vi "LineController Analogue init v3.0.vi"(0 "lines":tag="Dev2/ao0", 1 "Power level (0-1)":dbl=1.0 min=0.0 max=1.0, 3 "error in":errorcluster, 4 "Level at max (0-5V)":dbl=5.0 min=0.0 max=5.0 step=0.05) -> (5 "task out":refnum<k21>, 6 "Gauge":dbl(knob) scale=0.0..5.0, 7 "error out":errorcluster)   [LabVIEW 2014]
uses:
  <vilib>/DAQmx/create/channels.llb/DAQmx Create Channel (AO-Voltage-Basic).vi
  <vilib>/DAQmx/write.llb/DAQmx Write (Analog DBL 1Chan 1Samp).vi
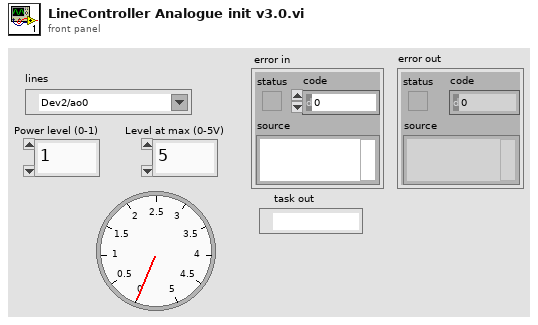
[diagram p1: front panel]
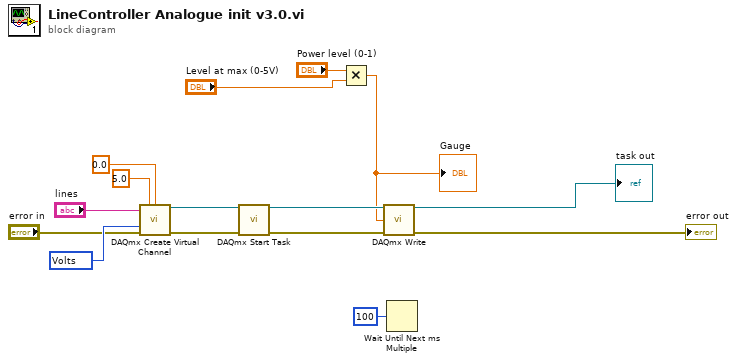
[diagram p0: block diagram]
diagram:
  w9 = 10348 items=["Volts"=10348, "From Custom Scale"=10065] ("units")
  n1 = call-poly <vilib>:"DAQmx Create Virtual Channel.vi"("maximum value"=5.0, "minimum value"=0.0, "physical channels"="lines", "units"=w9, "error in"="error in") -> ("task out"=w14:refnum<k21>, "error out"=w12:errorcluster)  [unwired: 9 in]
  n2 = call <vilib>:"DAQmx Start Task.vi"("task/channels in"=w14, "error in"=w12) -> ("task out"=w13:refnum<k21>, "error out"=w11:errorcluster)  [unwired: 12 in]
  n3 = Multiply(x="Power level (0-1)", y="Level at max (0-5V)") -> (x*y=w2:dbl)
  "Gauge" <- w2
  n4 = call-poly <vilib>:"DAQmx Write.vi"("task/channels in"=w13, "data"=w2, "error in"=w11) -> ("task out"=→"task out":refnum<k21>, "error out"=→"error out":errorcluster)  [unwired: 10 in, 1 out]
  n5 = Wait Until Next ms Multiple(millisecond multiple=u32 100) -> ()  [unwired: 1 out]
